vi "IZMoveAbs.vi"(0 "PRIORLib.IZIn":refnum<k7>, 1 "Location":dbl) -> (2 "PRIORLib.IZOut":refnum<k7>, 3 "error out":errorcluster, 4 "Return":i32)   [LabVIEW 2011]
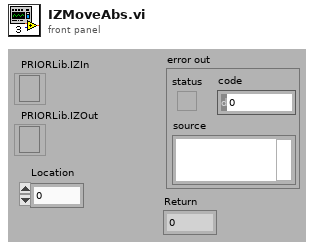
[diagram p1: front panel]
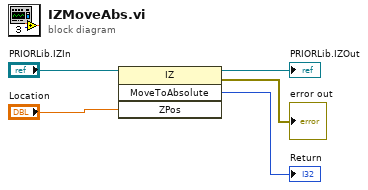
[diagram p0: block diagram]
diagram:
  n1 = invoke class="IZ" method="MoveToAbsolute"(reference="PRIORLib.IZIn", "ZPos"="Location") -> (reference out=→"PRIORLib.IZOut":refnum<k7>, error out=→"error out":errorcluster, "MoveToAbsolute"=→"Return":i32)  [unwired: 2 in, 1 out]
